vi "get_transitionTrigger.vi"(0 "HGF_DFSMVisitor":refnum<class "HGF_DFSMVisitor.lvclass">, 5 "error in (no error)":errorcluster) -> (14 "HGF_DFSMVisitor":refnum<class "HGF_DFSMVisitor.lvclass">, 16 "Trigger":T1, 17 "deviceVisitor":refnum<class "HGF_DeviceVisitor.lvclass">, 19 "error out":errorcluster)   [LabVIEW 2012, in "HGF_DeviceFSM.lvlib" / "HGF_DFSMVisitor.lvclass"]
doc: "This VI returns the HGF_DeviceFSM.lvsc transition trigger and device visitor."
uses:
  HGF_DFSMVisitor.lvclass
  HGF_DeviceFSM/HGF_DeviceFSM.lvsc/Trigger.ctl
  HGF_DeviceBaseClasses/HGF_DeviceVisitor/HGF_DeviceVisitor.lvclass
  HGF_DFSMVisitor.lvclass/HGF_DFSMVisitor.ctl
  HGF_DeviceFSM/HGF_DeviceFSM.lvsc
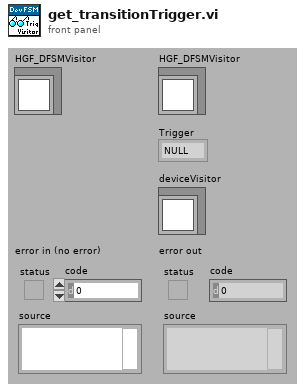
[diagram p1: front panel]
types:
  T1 = typedef "HGF_DeviceFSM.lvlib/HGF_DeviceFSM.lvsc/Trigger.ctl" = enum16{"NULL", "configure", "fault", "error", "resetError", "STOP", "visit", "not_configured", "done", "ok", "previsit", "configured"}
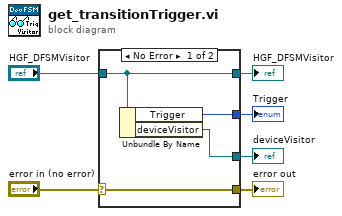
[diagram p0: block diagram]
diagram:
  n1 = case shown="No Error" "error in (no error)" {
    selector: "error in (no error)" -> [w10 w11]
    tunnel: [w10 w11] -> w5
    tunnel: [w7 w12] -> w3
    tunnel: "HGF_DFSMVisitor" -> [w7 w12]
    tunnel: [w8 _] -> w2
    tunnel: [w9 _] -> w1
    frame No Error {
      n2 = Unbundle By Name(w7) -> ("Trigger"=w8:T1, "deviceVisitor"=w9:refnum<class "HGF_DeviceVisitor.lvclass">)
    }
    frame Error {
    }
  }
  "error out" <- w5
  "HGF_DFSMVisitor" <- w3
  "Trigger" <- w2
  "deviceVisitor" <- w1
